vi "Disconnect.vi"(8 "error in (no error)":errorcluster, 10 "Disconnection list in":string, 11 "Mock NI-SWITCH Consumer in":refnum<class "Mock NI-SWITCH Consumer.lvclass">=refnum) -> (0 "error out":errorcluster, 3 "Mock NI-SWITCH Consumer out":refnum<class "Mock NI-SWITCH Consumer.lvclass">)   [LabVIEW 2020, in "Mock NI-SWITCH Consumer.lvclass"]
uses:
  Mock NI-SWITCH Consumer.lvclass
  Mock NI-SWITCH Consumer.lvclass/Mock NI-SWITCH Consumer.ctl
  NI-SWITCH Consumer/NI-SWITCH Consumer.lvclass
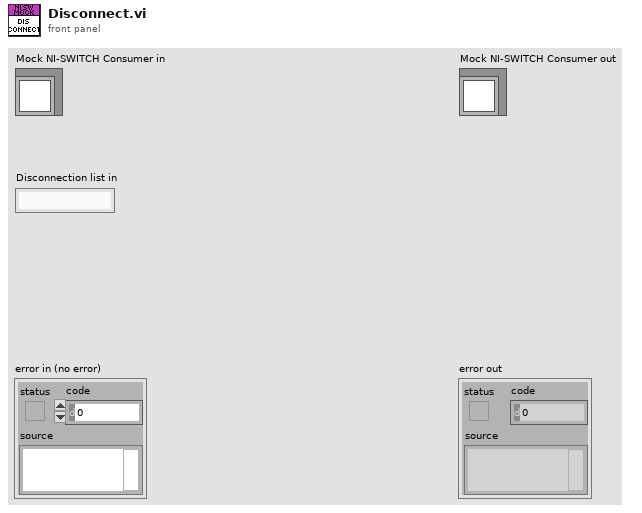
[diagram p1: front panel]
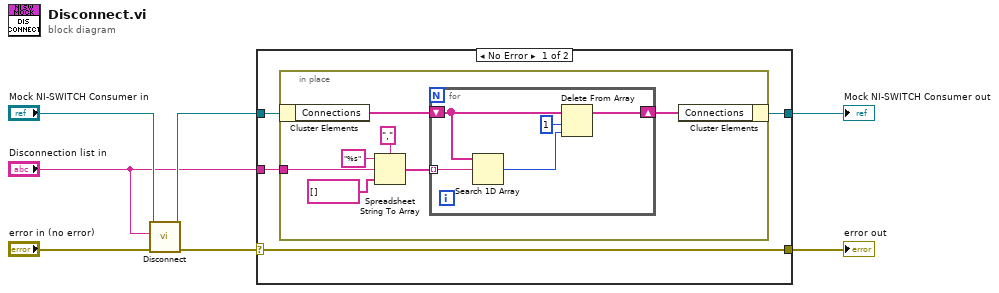
[diagram p0: block diagram]
diagram:
  n1 = call-parent "Disconnect.vi"("error in (no error)"="error in (no error)", "Disconnection list in"="Disconnection list in", "NI-SWITCH Consumer in"="Mock NI-SWITCH Consumer in") -> ("error out"=w5:errorcluster, "NI-SWITCH Consumer out"=w4:refnum<class "Mock NI-SWITCH Consumer.lvclass">)  [unwired: 7 in]
  n2 = case shown="No Error" w5 {
    selector: w5 -> [w8 w24]
    tunnel: w4 -> [w11 w25]
    tunnel: "Disconnection list in" -> [w10 _]
    tunnel: [w9 w25] -> w2
    tunnel: [w8 w24] -> w1
    frame No Error {
      n3 = in-place {
        in-place-border: w10 -> [w18]
        n4 = in-place-cluster #1(w11) -> ("Connections"=w14:string[])
        n5 = Spreadsheet String To Array(delimiter (Tab)=",", format string="%s", spreadsheet string=w18, array type (2D Dbl)=string[] [] ("Connections")) -> (array=w13:string[])
        n6 = for {
          shift-right: [w19] -> w12
          shift-left: w14 -> [w22]
          tunnel: w13 -> [w23] mode=indexing
          n7 = Search 1D Array(1D array=w22, element=w23) -> (index of element=w21:i32)  [unwired: 1 in]
          n8 = Delete From Array(array=w22, length=1, index=w21) -> (array with subset deleted=w19:string[])  [unwired: 1 out]
        }
        n9 = in-place-cluster #1("Connections"=w12) -> (w9:refnum<class "Mock NI-SWITCH Consumer.lvclass">)
      }
    }
    frame Error {
    }
  }
  "error out" <- w1
  "Mock NI-SWITCH Consumer out" <- w2
